vi "4bmilo.vi"() -> ()   [LabVIEW 2010]
uses:
  <vilib>/express/express arith-compare/Formula/XNode/ExpressFormulaBlockNode.xnode
  <vilib>/express/express shared/transition.llb/Dynamic To Waveform Array.vi
  <vilib>/express/express shared/transition.llb/Waveform Array To Dynamic.vi
  <vilib>/express/express arith-compare/Formula/Block/exnFormulaBlock how many pts in the wave.vi
  <vilib>/express/express shared/ex_Modify Signal Name.vi
  <vilib>/measure/NI_MABase.lvlib
panel:
  out "Pøenosová charakteristika":cluster{"Y":dbl[], "Y":dbl[]}[](graph)
  out "au(dB)":dbl
  out "Au":dbl
  out "f(Hz)":dbl
  out "Uin(V)":dbl
  out "Uout(V)":dbl
  out "Ugen=f(t)":waveform(dbl)(graph)
  out "fgen(Hz)":dbl=10.0 format="%0.2p"
  in  "fmax(Hz)":i32
  in  "krok":i32
  in  "fmin(Hz)":i32
  in  "Typ signálu":T1(ring)
  in  "Ugen(V)":dbl=1.0 format="%0.2p"
  # "Automatizovaný snímaè pøenosových charakteristik"
  # "Rozmítaný generátor"
  # "Snímaè charakteristik"
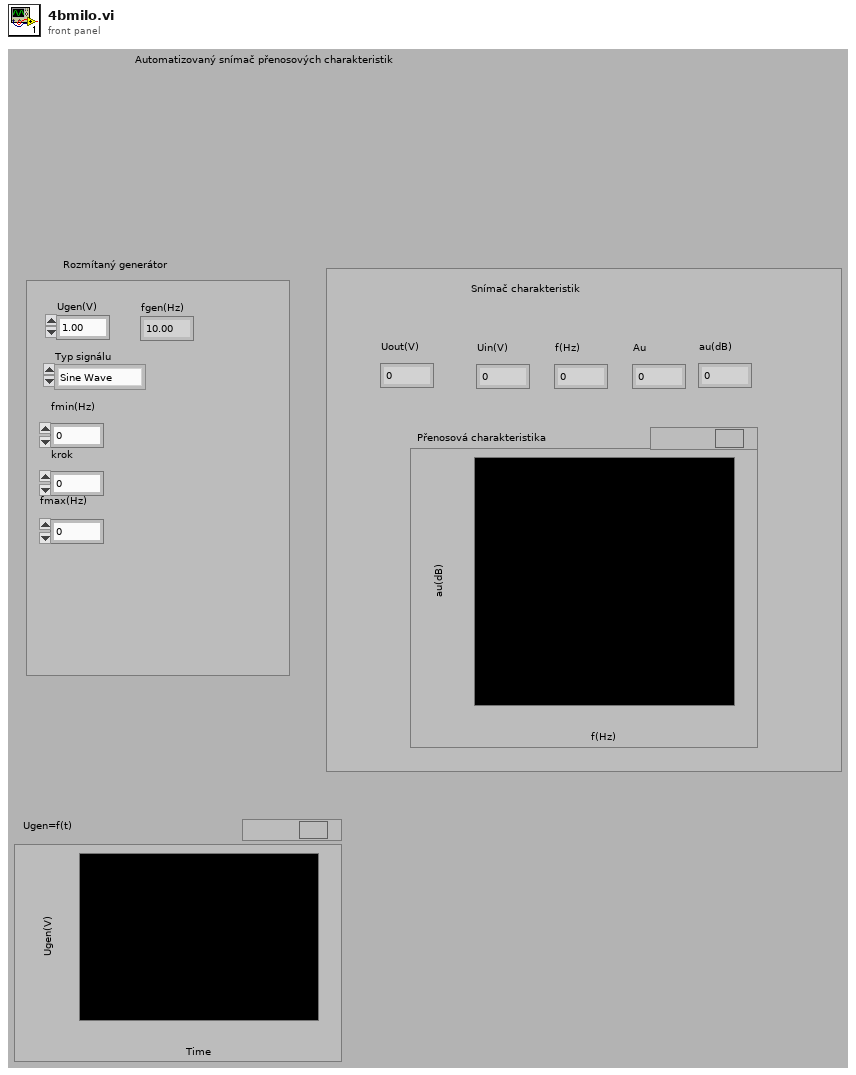
[diagram p1: front panel]
types:
  T1 = enum16{"Sine Wave", "Triangle Wave", "Square Wave", "Sawtooth Wave"}
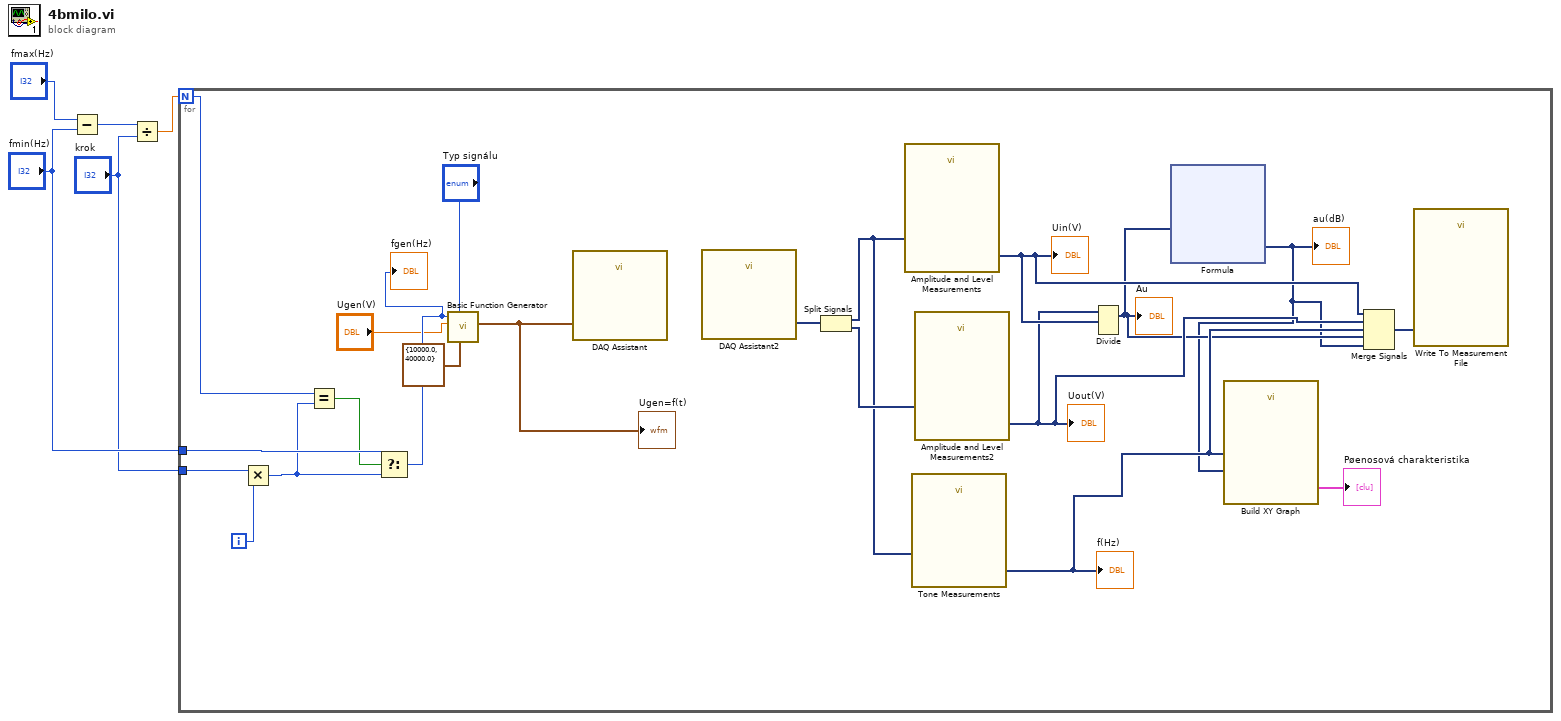
[diagram p0: block diagram]
diagram:
  n1 = Subtract(x="fmax(Hz)", y="fmin(Hz)") -> (x-y=w4:i32)
  n2 = Divide(x=w4, y="krok") -> (x/y=w3:dbl)
  n3 = for {
    N: w3 -> [w21]
    tunnel: "fmin(Hz)" -> [w23]
    tunnel: "krok" -> [w25]
    i -> [w24]
    n4 = Multiply(x=w25, y=w24) -> (x*y=w22:i32)
    n5 = Equal?(x=w21, y=w22) -> (x = y?=w20:bool)
    n6 = Select(t=w23, s=w20, f=w22) -> (s? t:f=w19:i32)
    "fgen(Hz)" <- w19
    n7 = call <vilib>:"Basic Function Generator.vi"("sampling info"=cluster{"Fs":dbl, "#s":dbl} {"Fs"=10000.0, "#s"=40000.0}, "signal type"="Typ signálu", "amplitude"="Ugen(V)", "frequency"=w19) -> ("signal out"=w17:waveform(dbl))  [unwired: 5 in, 2 out]
    "Ugen=f(t)" <- w17
    n8 = call "DAQ Assistant"("data"=w17) -> ()  [unwired: 17 in, 2 out]
    n9 = call "DAQ Assistant2"() -> ("data"=w15:dynamicdata)  [unwired: 17 in, 2 out]
    n10 = Split Signals(w15) -> (w13:dynamicdata, w14:dynamicdata)  [unwired: 2 in]
    n11 = call "Amplitude and Level Measurements"("Signals"=w13) -> ("RMS"=w10:dynamicdata)  [unwired: 13 in, 1 out]
    "Uin(V)" <- w10
    n12 = call "Tone Measurements"("Signals"=w13) -> ("Frequency"=w8:dynamicdata)  [unwired: 9 in, 1 out]
    "f(Hz)" <- w8
    n13 = call "Amplitude and Level Measurements2"("Signals"=w14) -> ("RMS"=w9:dynamicdata)  [unwired: 13 in, 1 out]
    "Uout(V)" <- w9
    n14 = Divide(1:w10, 2:w9) -> (0:w7:dynamicdata)  [unwired: 1 in, 1 out]
    "Au" <- w7
    n15 = xnode "Formula"("Au"=w7) -> ("Result"=w6:dynamicdata)  [unwired: 1 in, 1 out]
    "au(dB)" <- w6
    n16 = call "Build XY Graph"("Y Input"=w6, "X Input"=w8) -> ("XY Graph"=→"Pøenosová charakteristika":cluster{"Y":dbl[], "Y":dbl[]}[])  [unwired: 3 in, 6 out]
    n17 = Merge Signals(w10, w9, w8, w7, w6) -> (w11:dynamicdata)
    n18 = call "Write To Measurement File"("Signals"=w11) -> ()  [unwired: 16 in, 3 out]
  }
